vi "Is Open.vi"(8 "error in (no error)":errorcluster, 11 "TCP Server in":refnum<class "TCP Server.lvclass">) -> (0 "error out":errorcluster, 2 "Is Open":bool, 3 "TCP Server out":refnum<class "TCP Server.lvclass">)   [LabVIEW 2020, in "Stream-TCP.lvlib" / "TCP Server.lvclass"]
uses:
  TCP Server.lvclass
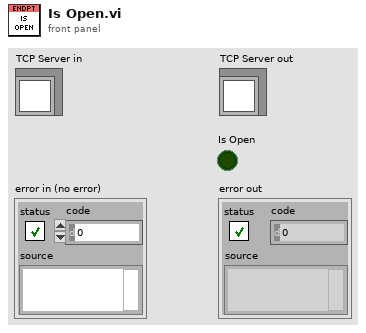
[diagram p1: front panel]
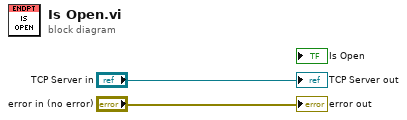
[diagram p0: block diagram]
diagram:
  "error out" <- "error in (no error)"
  "TCP Server out" <- "TCP Server in"
